vi "Read Power FIFO Direct Dispatch.vi"(8 "error in (no error)":errorcluster, 9 "Timeout (ms)":i32=100, 10 "Data in":T1[](array[typedef])=[{"measurement"=[], "dT"=0.0, "Timestamp"=0}, {"measurement"=[], "dT"=0.0, "Timestamp"=0}], 11 "CIFTag in":refnum<class "CIFChannels.lvclass">) -> (0 "error out":errorcluster, 1 "timed out?":bool, 2 "Data out":T1[](array[typedef]), 3 "CIFTag out":refnum<class "CIF_NIChn_Fifo_Power.lvclass">, 4 "Header":T2)   [LabVIEW 2021, in "CIF_NIChn_Fifo_Power.lvclass"]
uses:
  CIF_NIChn_Fifo_Power.lvclass
  CIFChannels/Typedef/Direction.ctl
  CIFChannels/CIFChannels.lvclass
  CIFChannels/Typedef/Channel State.ctl
  NIChn/CIF_NIChn.lvclass
  D:/dev/CIF-LVCore/src/Channels/CIF_NIChn/NIChn/CIF_NIChn.lvclass
  <vilib>/CIFChannels/CIFChannelCore.lvlib
  ChannelCommon/typedef/FIFO Header.ctl
  ChannelCommon/ChannelCommon.lvlib
  ChannelCommon/typedef/Datatype Waveform.ctl
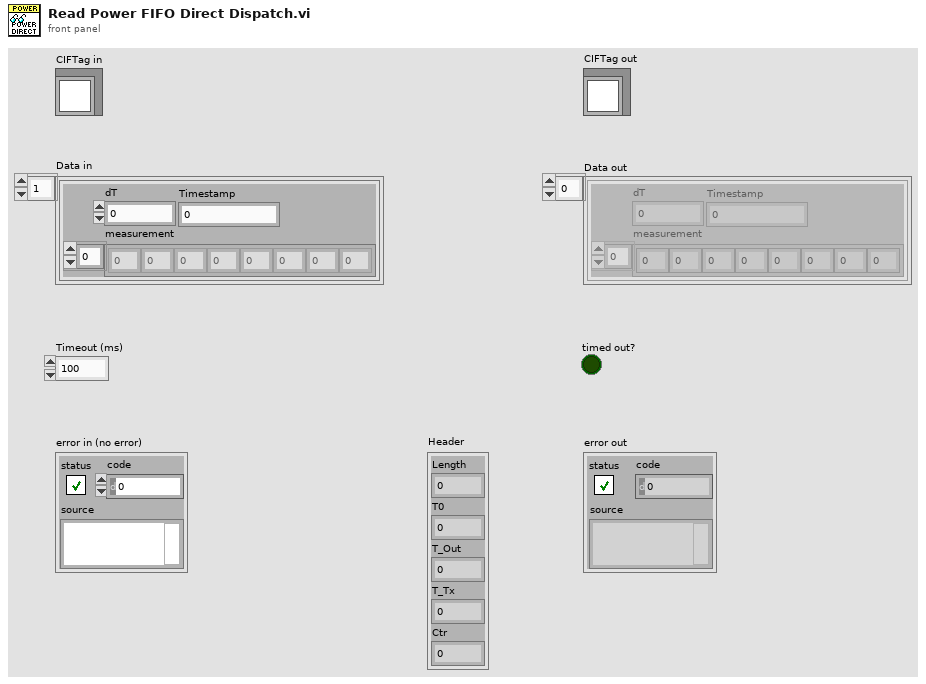
[diagram p1: front panel]
types:
  T1 = typedef "ChannelCommon.lvlib/Datatype Waveform.ctl" = cluster{"measurement":dbl[], "dT":dbl, "Timestamp":u64}
  T2 = typedef "ChannelCommon.lvlib/FIFO Header.ctl" = cluster{"Length":u64, "T0":u64, "T_Out":u64, "T_Tx":u64, "Ctr":u64}
  T3 = typedef "CIFChannels.lvclass/Channel State.ctl" = enum16{"Creating", "Disconnected", "Connecting", "Connected", "Destroyed"}
  T4 = typedef "CIFChannels.lvclass/Direction.ctl" = enum16{"Publisher", "Subscriber"}
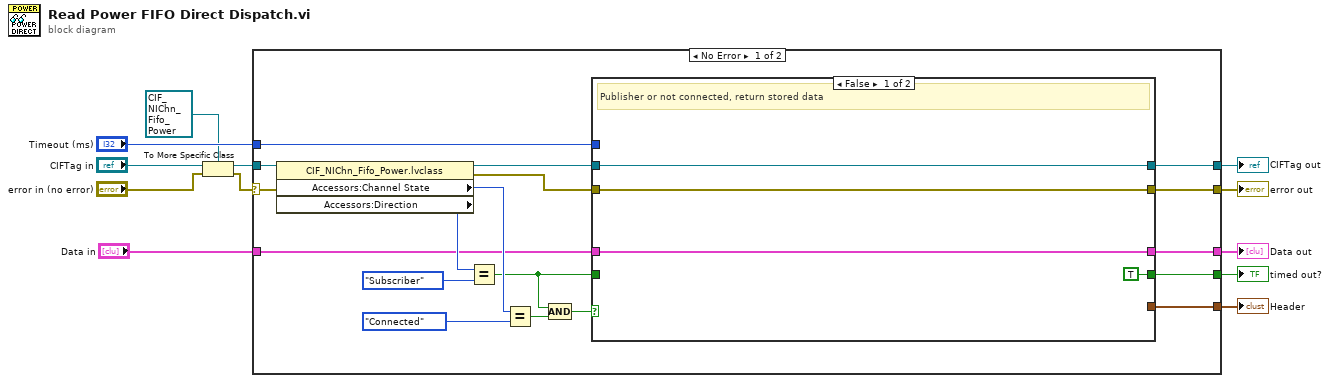
[diagram p0: block diagram]
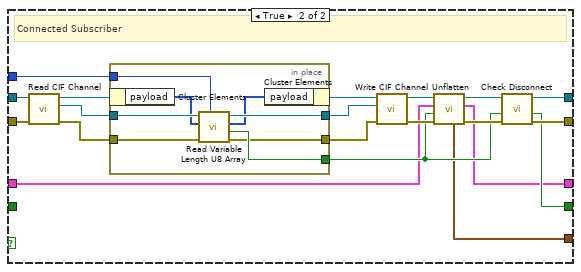
[diagram p2: hidden frame]
diagram:
  n1 = To More Specific Class(target class=refnum<class "CIF_NIChn_Fifo_Power.lvclass"> refnum ("CIFTag in"), reference="CIFTag in", error in="error in (no error)") -> (specific class reference=w5:refnum<class "CIF_NIChn_Fifo_Power.lvclass">, error out=w4:errorcluster)
  n2 = case shown="No Error" w4 {
    selector: w4 -> [w27 w65]
    tunnel: [w16 w65] -> w12
    tunnel: [w17 w64] -> w11
    tunnel: w5 -> [w28 w64]
    tunnel: [w30 _] -> w10
    tunnel: [w29 w63] -> w2
    tunnel: "Timeout (ms)" -> [w15 _]
    tunnel: [w14 _] -> w8
    tunnel: "Data in" -> [w13 w63]
    frame No Error {
      n3 = property class="CIF_NIChn_Fifo_Power.lvclass"(reference=w28, error in=w27) -> (reference out=w26:refnum<class "CIF_NIChn_Fifo_Power.lvclass">, error out=w25:errorcluster, "Accessors:Channel State"=w22:T3, "Accessors:Direction"=w24:T4)
      n4 = Equal?(x=w24, y=Direction."Subscriber") -> (x = y?=w18:bool)
      n5 = Equal?(x=w22, y=Channel_State."Connected") -> (x = y?=w20:bool)
      n6 = Compound Arithmetic op=AND(w18, w20) -> (w19:bool)
      n7 = case shown="False" w19 {
        tunnel: [TRUE ("timeout out") w44] -> w30
        tunnel: [w31 w37] -> w29
        tunnel: w25 -> [w33 w53]
        tunnel: w26 -> [w34 w54]
        tunnel: w18 -> [_ _]
        tunnel: [w34 w52] -> w17
        tunnel: [w33 w51] -> w16
        tunnel: w15 -> [_ w43]
        tunnel: [_ w36] -> w14
        tunnel: w13 -> [w31 w35]
        frame False {
          # "Publisher or not connected, return stored data"
        }
        frame True {
          # "Connected Subscriber"
          n8 = call "Read CIF Channel.vi"("error in (no error)"=w53, "CIFTag in"=w54) -> ("error out"=w48:errorcluster, "CIF Channel"=w49:refnum<k21>, "CIFTag out"=w50:refnum<class "CIF_NIChn_Fifo_Power.lvclass">)  [unwired: 7 in]
          n9 = in-place {
            in-place-border: [w60] -> w38
            in-place-border: w49 -> [w62]
            in-place-border: w48 -> [w61]
            in-place-border: [w59] -> w45
            in-place-border: [w58] -> w46
            in-place-border: w43 -> [w57]
            n10 = in-place-cluster #1(w50) -> ("payload"=w56:u8[])
            n11 = call <vilib>:"Read Variable Length U8 Array.vi"("Timeout (ms)"=w57, "error in"=w61, "Payload in"=w56, "CIF Channel in"=w62) -> ("error out"=w58:errorcluster, "Timed out?"=w60:bool, "Payload out"=w55:u8[], "CIF Channel out"=w59:refnum<k21>)  [unwired: 4 in]
            n12 = in-place-cluster #1("payload"=w55) -> (w47:refnum<class "CIF_NIChn_Fifo_Power.lvclass">)
          }
          n13 = call "Write CIF Channel.vi"("error in (no error)"=w46, "CIF Channel"=w45, "CIFTag in"=w47) -> ("error out"=w41:errorcluster, "CIFTag out"=w42:refnum<class "CIF_NIChn_Fifo_Power.lvclass">)  [unwired: 7 in]
          n14 = call "Unflatten.vi"("error in (no error)"=w41, "timeout in"=w38, "Data in"=w35, "CIFFifoCAN in"=w42) -> ("error out"=w39:errorcluster, "Data out"=w37:T1[], "CIFFifoCAN out"=w40:refnum<class "CIF_NIChn_Fifo_Power.lvclass">, "Header"=w36:T2)  [unwired: 4 in]
          n15 = call "Check Disconnect.vi"("error in (no error)"=w39, "timeout in"=w38, "CIFTag in"=w40) -> ("error out"=w51:errorcluster, "timeout out"=w44:bool, "CIFTag out"=w52:refnum<class "CIF_NIChn_Fifo_Power.lvclass">)  [unwired: 5 in, 1 out]
        }
      }
    }
    frame Error {
    }
  }
  "error out" <- w12
  "CIFTag out" <- w11
  "timed out?" <- w10
  "Header" <- w8
  "Data out" <- w2
